vi "SP Convert Display to Limit Format.vi"(4 "Display Format":T2=7 items=["Log Mag", "Phase", "Expanded Phase", "Delay", "Smith", "Polar", "Lin Mag", "SWR", "Loss", "Real", "Imaginary"], 5 "S Parameter":T3 caption="Parameter" {"Stimulus Port" min=1 step=1; "Response Port" min=1 step=1}) -> (1 "Limit Format":T1)   [LabVIEW 2011]
uses:
  TypeDefs/SP Parameter.ctl
  TypeDefs/SP Display Format.ctl
  TypeDefs/SP Format.ctl
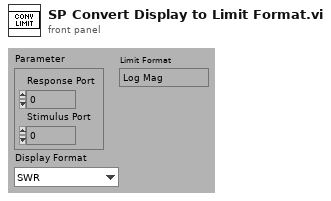
[diagram p1: front panel]
types:
  T1 = typedef "SP Format.ctl" = enum16{"Log Mag", "Lin Mag", "SWR", "Phase", "Expanded Phase", "Delay", "Insertion Loss", "Isolation", "Return Loss"}
  T2 = typedef "SP Display Format.ctl" = i32
  T3 = typedef "SP Parameter.ctl" = cluster{"Stimulus Port":i8, "Response Port":i8}
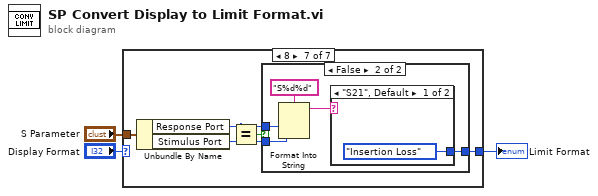
[diagram p0: block diagram]
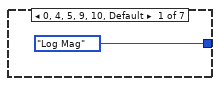
[diagram p2: hidden frame]
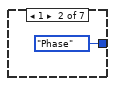
[diagram p3: hidden frame]
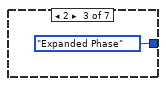
[diagram p4: hidden frame]
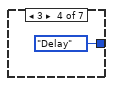
[diagram p5: hidden frame]
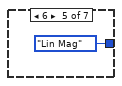
[diagram p6: hidden frame]
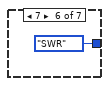
[diagram p7: hidden frame]
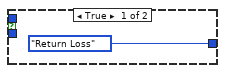
[diagram p8: hidden frame]
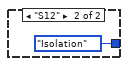
[diagram p9: hidden frame]
diagram:
  n1 = case shown="8" "Display Format" {
    tunnel: [SP_Format."Log Mag" ("Limit Format") SP_Format."Phase" ("Limit Format") SP_Format."Expanded Phase" ("Limit Format") SP_Format."Delay" ("Limit Format") SP_Format."Lin Mag" ("Limit Format") SP_Format."SWR" ("Limit Format") w14] -> w1
    tunnel: "S Parameter" -> [_ _ _ _ _ _ w13]
    frame 0, 4, 5, 9, 10, Default {
    }
    frame 1 {
    }
    frame 2 {
    }
    frame 3 {
    }
    frame 6 {
    }
    frame 7 {
    }
    frame 8 {
      n2 = Unbundle By Name(w13) -> ("Response Port"=w11:i8, "Stimulus Port"=w10:i8)
      n3 = Equal?(x=w11, y=w10) -> (x = y?=w12:bool)
      n4 = case shown="False" w12 {
        tunnel: [SP_Format."Return Loss" ("Limit Format") w20] -> w14
        tunnel: w11 -> [_ w18]
        tunnel: w10 -> [_ w17]
        frame True {
        }
        frame False {
          n5 = Format Into String(format string="S%d%d", w18, w17) -> (resulting string=w16:string)  [unwired: 2 in, 1 out]
          n6 = case shown="\"S21\", Default" w16 {
            tunnel: [SP_Format."Insertion Loss" ("Limit Format") SP_Format."Isolation" ("Limit Format")] -> w20
            frame "S21", Default {
            }
            frame "S12" {
            }
          }
        }
      }
    }
  }
  "Limit Format" <- w1
